vi "ICNC Wait Input State Buf.vi"(6 "ClearBufferIfError":i32, 7 "LockIfError":i32, 8 "error in (no error)":errorcluster caption="entrée d'erreur (pas d'erreur)", 9 "TimeOut":u32, 10 "InputValue":i32, 11 "InputNo":u32) -> (0 "error out":errorcluster caption="sortie d'erreur", 3 "function return":u32)   [LabVIEW 2012, in "ICNC2.lvlib"]
doc: "DWORD ICNC_WaitInputStateBuf(DWORD InputNo,\n BOOL InputValue,\n DWORD TimeOut,\n BOOL LockIfError=FALSE,\n BOOL ClearBufferIfError = FALSE);"
uses:
  <userlib>/ICNC/ICNC2.lvlib
  <userlib>/ICNC/ICNC2.dll
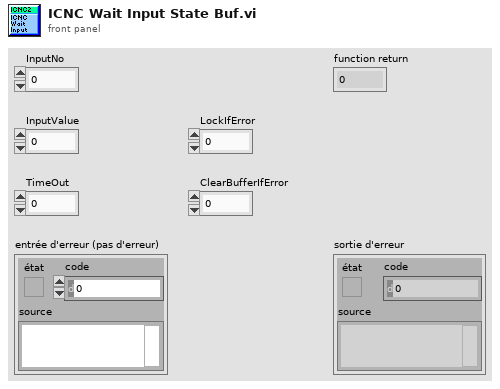
[diagram p1: front panel]
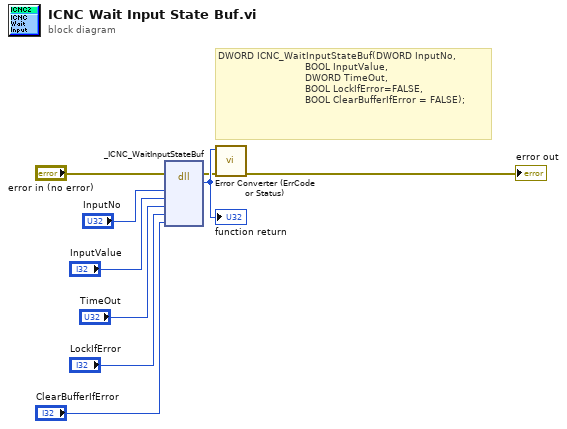
[diagram p0: block diagram]
diagram:
  # "DWORD ICNC_WaitInputStateBuf(DWORD InputNo,\n                             BOOL InputValue,\n                             DWORD TimeOut,\n                             BOOL LockIfError=FALSE,\n                             BOOL ClearBufferIfError = FALSE);"
  n1 = dll-call lib="C:/Program Files (x86)/National Instruments/LabVIEW 2012/user.lib/ICNC/ICNC2.*" fn="_ICNC_WaitInputStateBuf"(error in="error in (no error)", "InputNo"="InputNo", "InputValue"="InputValue", "TimeOut"="TimeOut", "LockIfError"="LockIfError", "ClearBufferIfError"="ClearBufferIfError") -> (error out=w2:errorcluster, w9:u32)  [unwired: 7 in, 1 out]
  "function return" <- w9
  n2 = call <userlib>:"Error Converter (ErrCode or Status).vi"("error in (no error)"=w2, "error code"=w9) -> ("error out"=→"error out":errorcluster)  [unwired: 9 in]
